vi "Moving_Average (SubVI).vi"(10 "Waveform":waveform(dbl), 11 "Moving Average Width":i32) -> (2 "x/y":dbl, 3 "output waveform":waveform(dbl)(graph))   [LabVIEW 2016]
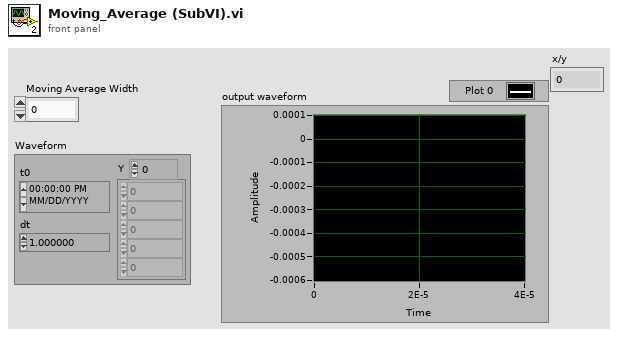
[diagram p1: front panel]
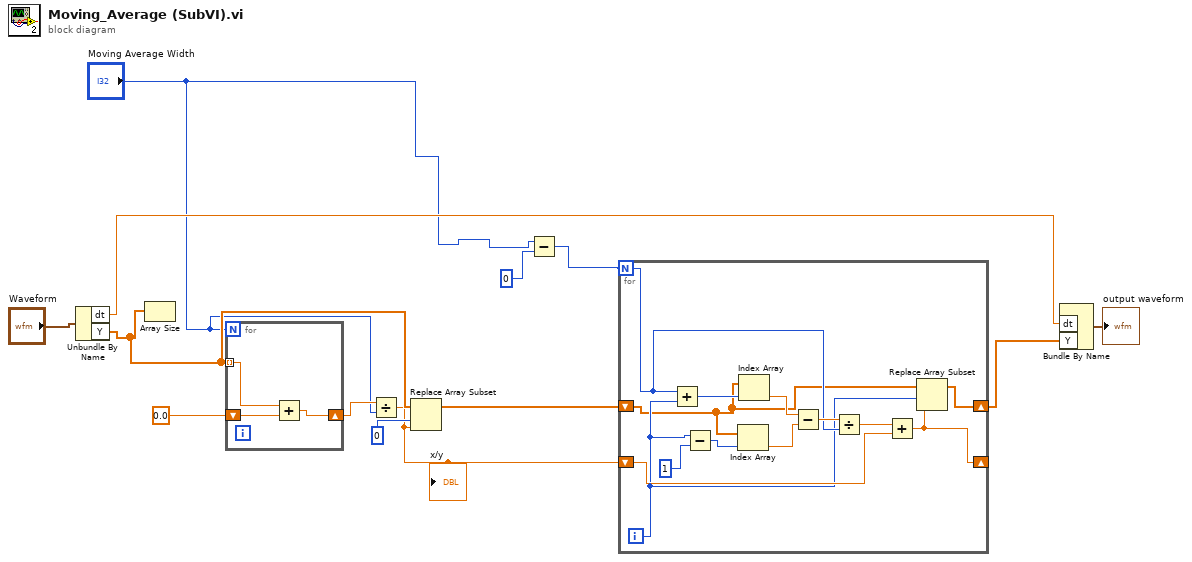
[diagram p0: block diagram]
diagram:
  n1 = Unbundle By Name("Waveform") -> ("dt"=w2:dbl, "Y"=w8:dbl[])
  n2 = Array Size(array=w8) -> ()  [unwired: 1 out]
  n3 = for {
    N: "Moving Average Width" -> [_]
    tunnel: w8 -> [w16] mode=indexing
    shift-right: [w14] -> w10
    shift-left: 0.0 -> [w15]
    n4 = Add(x=w16, y=w15) -> (x+y=w14:dbl)
  }
  n5 = Divide(x=w10, y="Moving Average Width") -> (x/y=w4:dbl)
  "x/y" <- w4
  n6 = Replace Array Subset(array=w8, new element=w4, index=0) -> (w5:dbl[])
  n7 = Subtract(x="Moving Average Width", y=0) -> (x-y=w6:i32)
  n8 = for {
    N: w6 -> [w23]
    shift-right: [w17] -> w3
    shift-left: w5 -> [w18]
    shift-right: [w20] -> _
    shift-left: w4 -> [w21]
    i -> [w19]
    n9 = Add(x=w23, y=w19) -> (x+y=w29:i32)
    n10 = Subtract(x=w19, y=1) -> (x-y=w27:i32)
    n11 = Index Array(array=w18, index=w27) -> (element=w25:dbl)
    n12 = Index Array(array=w18, index=w29) -> (element=w26:dbl)
    n13 = Subtract(x=w26, y=w25) -> (x-y=w24:dbl)
    n14 = Divide(x=w24, y=w23) -> (x/y=w22:dbl)
    n15 = Add(x=w22, y=w21) -> (x+y=w20:dbl)
    n16 = Replace Array Subset(array=w18, new element=w20, index=w19) -> (w17:dbl[])
  }
  n17 = Bundle By Name("dt"=w2, "Y"=w3) -> (→"output waveform":waveform(dbl))  [unwired: 1 in]
